vi "Append Port To Source Host.vi"(0 "message in":T1, 5 "source port":u16, 7 "source address":u32, 11 "error in":errorcluster) -> (4 "message out":T1, 15 "error out":errorcluster)   [LabVIEW 2013, in "AMC.lvlib"]
uses:
  AMC.lvlib
  Message.ctl
  <vilib>/NI/Tools/Keyed Array/KeyedArray.ctl
  <vilib>/NI/Tools/Keyed Array/Tools_KeyedArray.lvlib
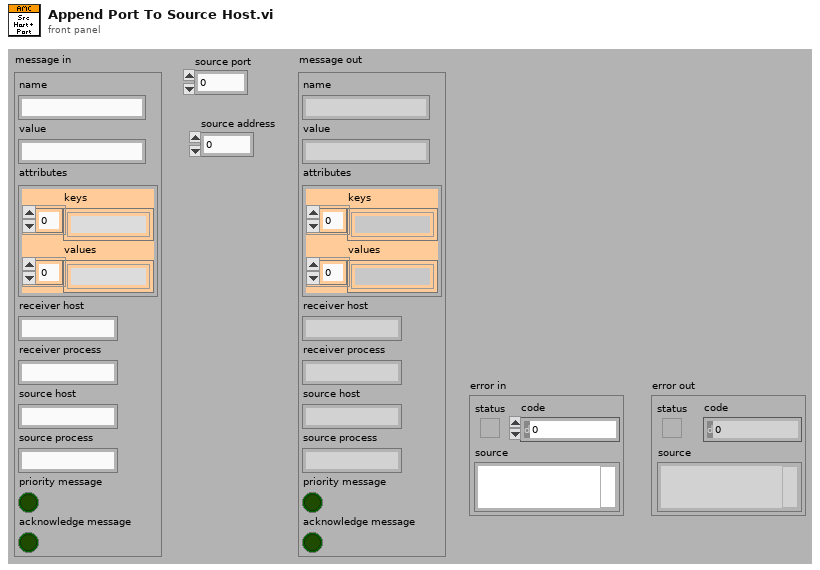
[diagram p1: front panel]
types:
  T1 = typedef "AMC.lvlib/Message.ctl" = cluster{"name":string, "value":string, "attributes":T2, "receiver host":string, "receiver process":string, "source host":string, "source process":string, "priority message":bool, "acknowledge message":bool}
  T2 = typedef "Tools_KeyedArray.lvlib/KeyedArray.ctl" = cluster{"keys":string[], "values":string[]}
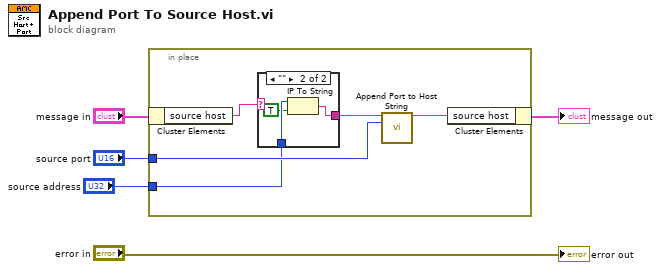
[diagram p0: block diagram]
diagram:
  n1 = in-place {
    in-place-border: "source port" -> [w9]
    in-place-border: "source address" -> [w6]
    n2 = in-place-cluster #1("message in") -> ("source host"=w8:string)
    n3 = case shown="\"\"" w8 {
      selector: w8 -> [w11 _]
      tunnel: [w11 w14] -> w7
      tunnel: w6 -> [_ w13]
      frame Default {
      }
      frame "" {
        n4 = IP To String(1:TRUE ("dot notation? (F)"), 2:w13) -> (0:w14:string)
      }
    }
    n5 = call "Append Port to Host String.vi"("host in"=w7, "port"=w9) -> ("host out"=w10:string)  [unwired: 13 in]
    n6 = in-place-cluster #1("source host"=w10) -> (→"message out":T1)
  }
  "error out" <- "error in"
